vi "Reset devices.vi"(8 "error in (no error)":errorcluster, 11 "FCR Mod ID":i32) -> (0 "error out":errorcluster)   [LabVIEW 2020]
uses:
  Newport_FCR100/Libraries/FCR100/Support/Device state -- enum.ctl
  Newport_FCR100/Libraries/FCR100/FCR100.lvlib
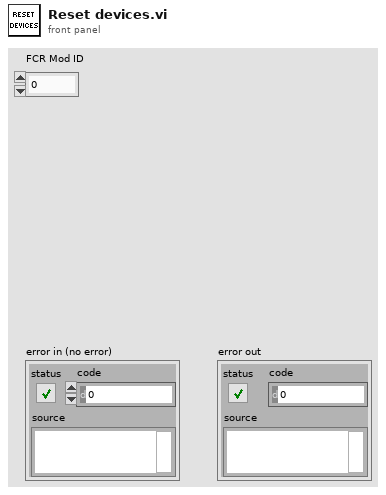
[diagram p1: front panel]
types:
  T1 = typedef "FCR100.lvlib/Device state -- enum.ctl" = enum16{"Not referenced", "Configuration", "Disable", "Ready", "Homing", "Motion"}
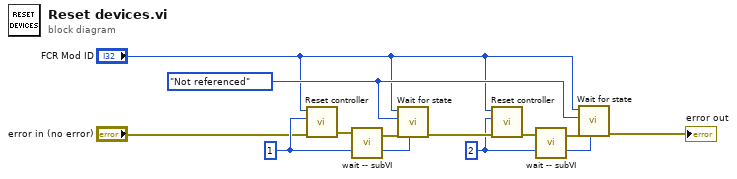
[diagram p0: block diagram]
diagram:
  w10 = Device_state_--_enum."Not referenced" ("State")
  w8 = u8 2 ("Address")
  w9 = u8 1 ("Address")
  n1 = call "Reset controller.vi"("error in"="error in (no error)", "Address"=w9, "Module ID"="FCR Mod ID") -> ("error out"=w4:errorcluster)  [unwired: 8 in]
  n2 = call "wait -- subVI.vi"("error in (no error)"=w4) -> ("error out"=w3:errorcluster)  [unwired: 4 in]
  n3 = call "Wait for state.vi"("Address"=w9, "error in (no error)"=w3, "State"=w10, "FCR Mod ID"="FCR Mod ID") -> ("error out"=w11:errorcluster)  [unwired: 6 in, 1 out]
  n4 = call "Reset controller.vi"("error in"=w11, "Address"=w8, "Module ID"="FCR Mod ID") -> ("error out"=w2:errorcluster)  [unwired: 8 in]
  n5 = call "wait -- subVI.vi"("error in (no error)"=w2) -> ("error out"=w1:errorcluster)  [unwired: 4 in]
  n6 = call "Wait for state.vi"("Address"=w8, "error in (no error)"=w1, "State"=w10, "FCR Mod ID"="FCR Mod ID") -> ("error out"=→"error out":errorcluster)  [unwired: 6 in, 1 out]
